vi "Drag & Drop Run Multi.vi"(0 "References In":T2(array[cluster]), 3 "error in":errorcluster) -> (6 "References Out":T2(array[cluster]), 9 "error out":errorcluster)   [LabVIEW 2015]
uses:
  <vilib>/Utility/miscctls.llb/LVPoint32TypeDef.ctl
panel:
  in  "Coords":T1[](array[typedef])
  out "Mouse Down?":bool[](array[boolean])
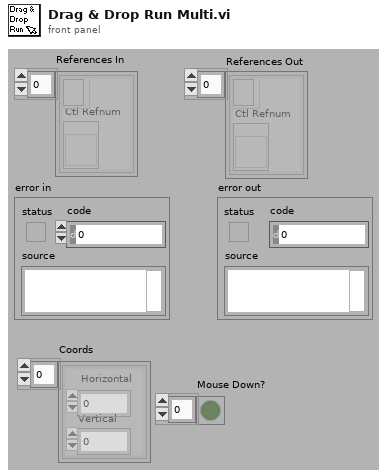
[diagram p1: front panel]
types:
  T1 = typedef "LVPoint32TypeDef.ctl" = cluster{"Horizontal":i32, "Vertical":i32}
  T2 = cluster{"Event Registration Refnum":refnum<event-registration>, "Ctl Refnum":refnum<vi>}[]
  T3 = typedef "LVPositionTypeDef.ctl" = cluster{"Left":i32, "Top":i32}
  T4 = cluster{"Event Registration Refnum":refnum<event-registration>, "Ctl Refnum":refnum<vi>}
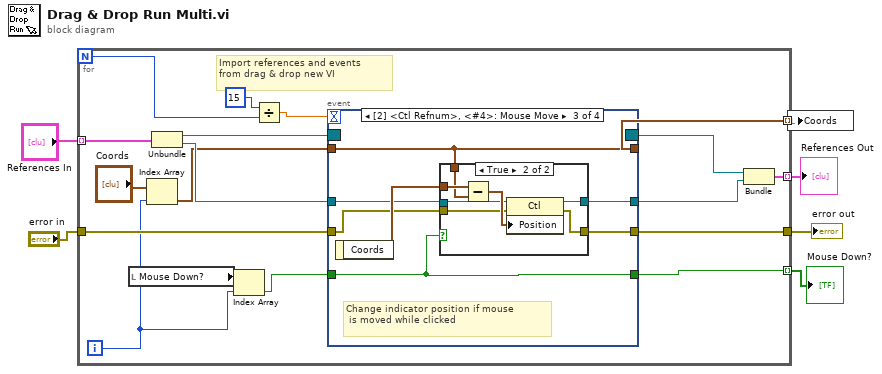
[diagram p0: block diagram]
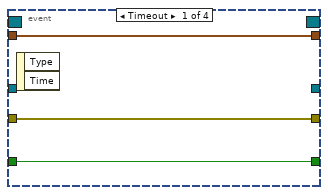
[diagram p2: hidden frame]
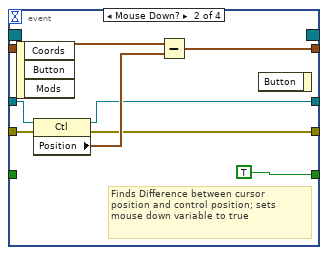
[diagram p3: hidden frame]
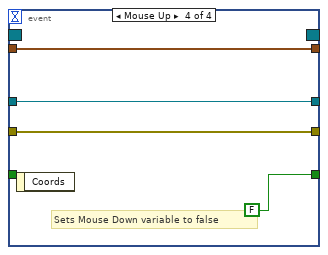
[diagram p5: hidden frame]
diagram:
  n1 = for {
    N -> [w8]
    tunnel: [w20] -> w6
    tunnel: [w19] -> w4 mode=indexing
    tunnel: "References In" -> [w18] mode=indexing
    tunnel: [w17] -> w3 mode=indexing
    tunnel: [w16] -> w2 mode=indexing
    tunnel: "error in" -> [w15]
    i -> [w12]
    # "Import references and events\nfrom drag & drop new VI"
    n2 = local read "Mouse Down?"() -> (w11:bool[])
    n3 = Index Array(array="Coords", index=w12) -> (element=w13:T1)
    n4 = Unbundle(w18) -> ("Event Registration Refnum"=w24:refnum<event-registration>, "Ctl Refnum"=w23:refnum<vi>)
    n5 = Index Array(array=w11, index=w12) -> (element=w10:bool)
    n6 = Divide(x=15, y=w8) -> (x/y=w7:dbl)
    n7 = event shown="[2] <Ctl Refnum>, <#4>: Mouse Move" {
      selector: w24 -> [_ _ _ _]
      dyn-events: [_ _ _ _] -> w22
      timeout: w7 -> [_ _ _ _]
      tunnel: w13 -> [w27 _ w41 w54]
      tunnel: [w27 w34 w41 w54] -> w16
      tunnel: [w25 TRUE ("Boolean") w36 FALSE ("Boolean")] -> w17
      tunnel: [_ w28 w40 w52] -> w21
      tunnel: w23 -> [_ w31 w39 w52]
      tunnel: w15 -> [w26 w30 w38 w53]
      tunnel: [w26 w29 w37 w53] -> w20
      tunnel: w10 -> [w25 _ w36 _]
      event Timeout {
        n8 = event-data() -> ()  [unwired: 3 out]
      }
      event Mouse Down? {
        # "Finds Difference between cursor\nposition and control position; sets\nmouse down variable to true"
        n9 = event-data() -> ("Coords"=w35:T1)  [unwired: 3 out]
        n10 = property class="Ctl"(reference=w31, error in=w30) -> (reference out=w28:refnum<vi>, error out=w29:errorcluster, "Position"=w32:T3)
        n11 = Subtract(x=w35, y=w32) -> (x-y=w34:T1)
        n12 = event-data() -> ()  [unwired: 1 in, 2 out]
      }
      event Mouse Move {
        # "Change indicator position if mouse\n is moved while clicked"
        n13 = event-data() -> ("Coords"=w42:T1)  [unwired: 1 out]
        n14 = case shown="True" w36 {
          tunnel: w42 -> [_ w51]
          tunnel: w41 -> [_ w50]
          tunnel: [w44 w48] -> w40
          tunnel: w39 -> [w44 w47]
          tunnel: w38 -> [w43 w46]
          tunnel: [w43 w45] -> w37
          frame False {
          }
          frame True {
            n15 = Subtract(x=w51, y=w50) -> (x-y=w49:T1)
            n16 = property class="Ctl"(reference=w47, error in=w46, "Position"=w49) -> (reference out=w48:refnum<vi>, error out=w45:errorcluster)
          }
        }
      }
      event Mouse Up {
        # "Sets Mouse Down variable to false"
        n17 = event-data() -> ()  [unwired: 2 out]
      }
    }
    n18 = Bundle("Event Registration Refnum"=w22, "Ctl Refnum"=w21) -> (w19:T4)  [unwired: 1 out]
  }
  "error out" <- w6
  "References Out" <- w4
  "Mouse Down?" <- w3
  n19 = local write "Coords"(w2) -> ()
